vi "Get Delimiter.vi"(8 "error in (no error)":errorcluster) -> (0 "error out":errorcluster, 2 "Namespace Delimiter":string)   [LabVIEW 2020, in "Tag Engine Core.lvlib" / "Tag Core.lvclass"]
doc: "_SubVI_"
uses:
  Tag Core.lvclass
  Tag Core.lvclass/Tag Core.ctl
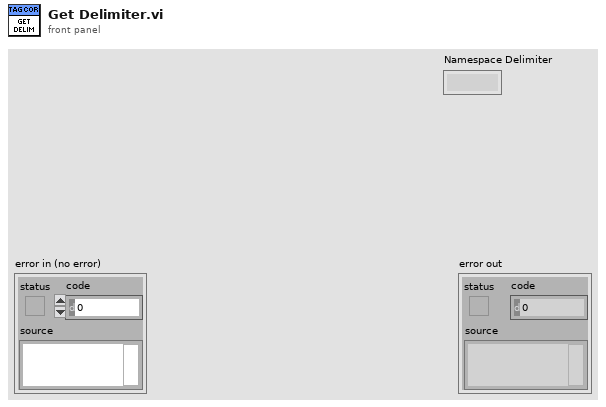
[diagram p1: front panel]
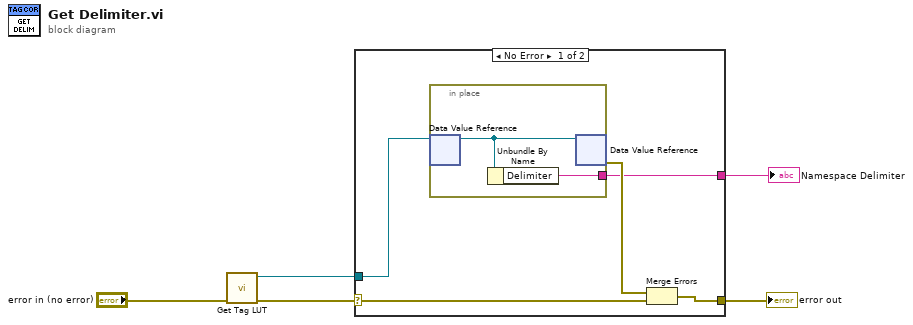
[diagram p0: block diagram]
diagram:
  n1 = call "Get Tag LUT.vi"("error in (no error)"="error in (no error)") -> ("error out"=w3:errorcluster, "Tag LUT Out"=w2:refnum<data-value>)  [unwired: 9 in]
  n2 = case shown="No Error" w3 {
    selector: w3 -> [w9 w13]
    tunnel: [w8 w13] -> w5
    tunnel: w2 -> [w10 _]
    tunnel: [w6 _] -> w1
    frame No Error {
      n3 = in-place {
        in-place-border: [w11] -> w6
        n4 = in-place-dvr #1(w10) -> (w12:refnum<class "Tag Core.lvclass">)  [unwired: 1 out]
        n5 = Unbundle By Name(w12) -> ("Delimiter"=w11:string)
        n6 = in-place-dvr #1(w12) -> (w7:errorcluster)  [unwired: 1 out]
      }
      n7 = Merge Errors(w7, w9) -> (w8:errorcluster)
    }
    frame Error {
    }
  }
  "error out" <- w5
  "Namespace Delimiter" <- w1
